vi "Replace with Nan.vi"(1 "Drives IN":T1(array[cluster])) -> (0 "Map":map{string, dbl}(c390))   [LabVIEW 2024, in "EtherCAT Model.lvlib"]
uses:
  EtherCAT Model.lvlib
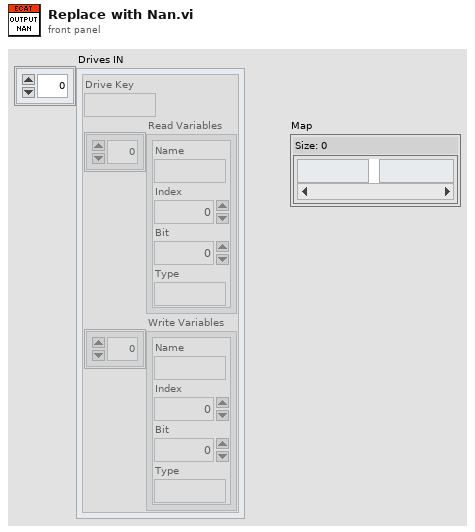
[diagram p1: front panel]
types:
  T1 = cluster{"Drive Key":string, "Read Variables":cluster{"Name":string, "Index":i32, "Bit":u8, "Type":string}[], "Write Variables":cluster{"Name":string, "Index":i32, "Bit":u8, "Type":string}[]}[]
  T2 = cluster{"Name":string, "Index":i32, "Bit":u8, "Type":string}[]
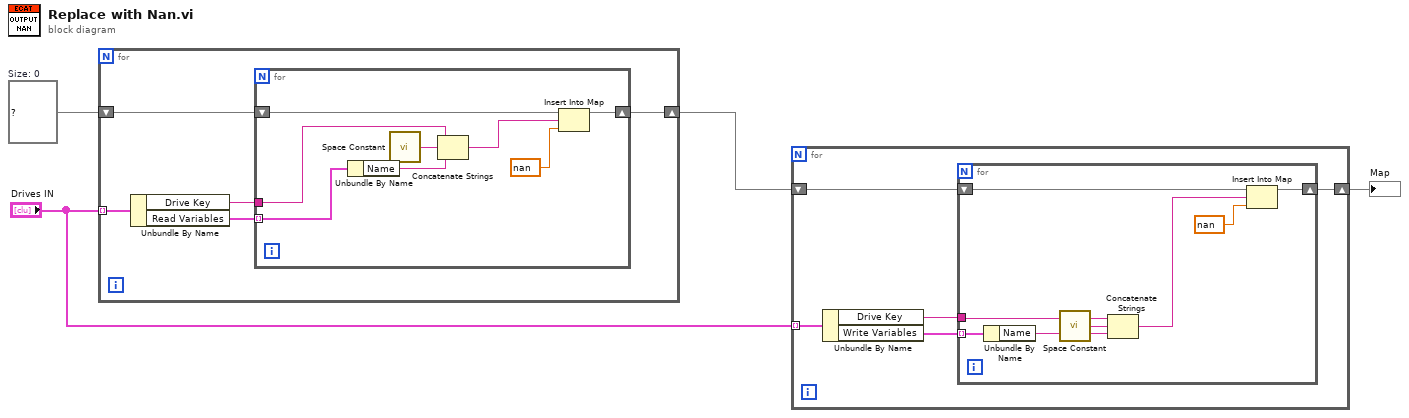
[diagram p0: block diagram]
diagram:
  w4 = map{string, dbl} {}  # Size: 0
  n1 = for {
    tunnel: "Drives IN" -> [w9] mode=indexing
    shift-right: [w5] -> w2
    shift-left: w4 -> [w7]
    n2 = Unbundle By Name(w9) -> ("Drive Key"=w6:string, "Read Variables"=w8:T2)
    n3 = for {
      tunnel: w8 -> [w16] mode=indexing
      tunnel: w6 -> [w15]
      shift-right: [w14] -> w5
      shift-left: w7 -> [w17]
      n4 = Unbundle By Name(w16) -> ("Name"=w13:string)
      n5 = call <vilib>:"Space Constant.vi"() -> ("String"=w12:string)
      n6 = Concatenate Strings(w15, w12, w13) -> (w11:string)
      n7 = Insert Into Map(map in=w17, key=w11, value=nan) -> (map out=w14:map{string, dbl})  [unwired: 2 out]
    }
  }
  n8 = for {
    tunnel: "Drives IN" -> [w22] mode=indexing
    shift-right: [w18] -> w3
    shift-left: w2 -> [w20]
    n9 = Unbundle By Name(w22) -> ("Drive Key"=w19:string, "Write Variables"=w21:T2)
    n10 = for {
      tunnel: w21 -> [w30] mode=indexing
      shift-right: [w26] -> w18
      shift-left: w20 -> [w27]
      tunnel: w19 -> [w28]
      n11 = Unbundle By Name(w30) -> ("Name"=w29:string)
      n12 = call <vilib>:"Space Constant.vi"() -> ("String"=w25:string)
      n13 = Concatenate Strings(w28, w25, w29) -> (w24:string)
      n14 = Insert Into Map(map in=w27, key=w24, value=nan) -> (map out=w26:map{string, dbl})  [unwired: 2 out]
    }
  }
  "Map" <- w3
